vi "Ease to a Stop.vi"() -> ()   [LabVIEW 2011, in "Sliding Menu Library.lvlib" / "Sliding Menu XControl.xctl"]
uses:
  Sliding Menu xControl/Sliding Menu XControl.xctl
panel:
  out "error out":errorcluster
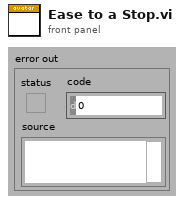
[diagram p1: front panel]
types:
  T1 = typedef "Sliding Menu Library.lvlib/Sliding Menu XControl.xctl/Sliding Menu State.ctl" = cluster{"Numeric":dbl, "Array of Button References":refnum<vi>[], "Space Between Menu Buttons":i32, "Number of Menu Buttons":i32, "Array of Button Names":string[], "Most Recent Vertical Position":i32, "This VI":refnum<vi>, "Current Action":T2, "Most Recent Distance Traveled":i32, "Method":T3, "Data In":T4}
  T2 = typedef "Sliding Menu Library.lvlib/Current User Action.ctl" = enum16{"Not Moving", "Mouse Down", "Mouse Up No Dragging", "Bounce Up Needed", "Bounce Down Needed", "Dragging", "Easing"}
  T3 = typedef "Sliding Menu Methods.ctl" = enum16{"Resize", "Move Up", "Move Down", "Move to 0"}
  T4 = typedef "Sliding Menu Library.lvlib/Sliding Menu XControl.xctl/Sliding Menu Data.ctl" = i32
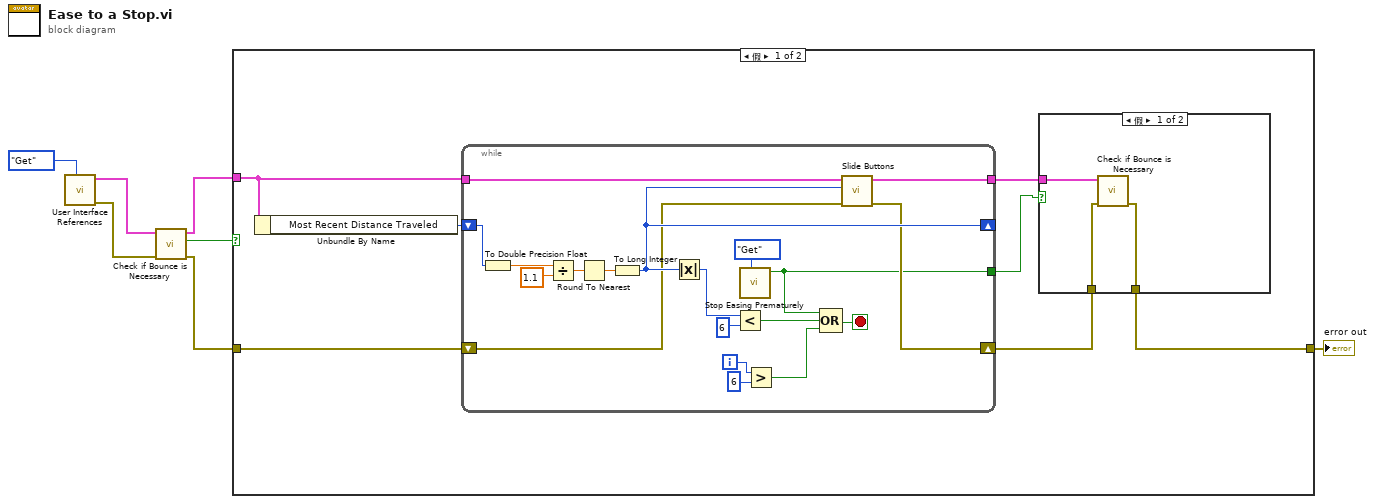
[diagram p0: block diagram]
diagram:
  n1 = call "User Interface References.vi"("Set or Get Value"=enum16{"Set", "Get"}."Get") -> ("error out"=w5:errorcluster, "Display State Out"=w6:T1)  [unwired: 9 in]
  n2 = call "Check if Bounce is Necessary.vi"("error in"=w5, "Display State In"=w6) -> ("error out"=w2:errorcluster, "Was Bounce Done?"=w4:bool, "Display State Out 2"=w3:T1)  [unwired: 7 in]
  n3 = case shown="假" w4 {
    tunnel: w3 -> [w14 _]
    tunnel: w2 -> [w12 w38]
    tunnel: [w9 w38] -> w1
    frame False {
      n4 = Unbundle By Name(w14) -> ("Most Recent Distance Traveled"=w13:i32)
      n5 = while {
        tunnel: w14 -> [w37]
        shift-right: [w24] -> w10
        shift-left: w12 -> [w20]
        shift-right: [w29] -> _
        shift-left: w13 -> [w30]
        tunnel: [w21] -> w11
        tunnel: [w19] -> w8
        i -> [w27]
        stop <- w25 stop-if-true
        n6 = To Double Precision Float(number=w30) -> (double precision float=w36:dbl)
        n7 = Divide(x=w36, y=1.1) -> (x/y=w31:dbl)
        n8 = Round To Nearest(number=w31) -> (nearest integer value=w32:dbl)
        n9 = To Long Integer(number=w32) -> (32bit integer=w29:i32)
        n10 = Absolute Value(x=w29) -> (abs(x)=w33:i32)
        n11 = Less?(x=w33, y=6) -> (x < y?=w26:bool)
        n12 = call "Stop Easing Prematurely.vi"("Set or Get Value"=enum16{"Set", "Get"}."Get") -> ("Stop?"=w19:bool)  [unwired: 10 in]
        n13 = Greater?(x=w27, y=6) -> (0:w22:bool)
        n14 = Compound Arithmetic op=OR(w19, w26, w22) -> (w25:bool)
        n15 = call "Slide Buttons.vi"("error in (no error)"=w20, "Distance"=w29, "Display State In"=w37) -> ("error out"=w24:errorcluster, "Display State Out"=w21:T1)  [unwired: 7 in]
      }
      n16 = case shown="假" w8 {
        tunnel: w11 -> [w17 _]
        tunnel: w10 -> [w16 w18]
        tunnel: [w15 w18] -> w9
        frame False {
          n17 = call "Check if Bounce is Necessary.vi"("error in"=w16, "Display State In"=w17) -> ("error out"=w15:errorcluster)  [unwired: 7 in, 2 out]
        }
        frame True {
        }
      }
    }
    frame True {
    }
  }
  "error out" <- w1
